vi "mediaBalls_v2.vi"(11 "Array Ball Pose + CamID":T1(array[cluster])) -> (3 "Ball out":cluster{"x":dbl, "y":dbl})   [LabVIEW 2018]
panel:
  in  "cluster":cluster{"x":dbl, "y":dbl}
  in  "Field Size 2":T2
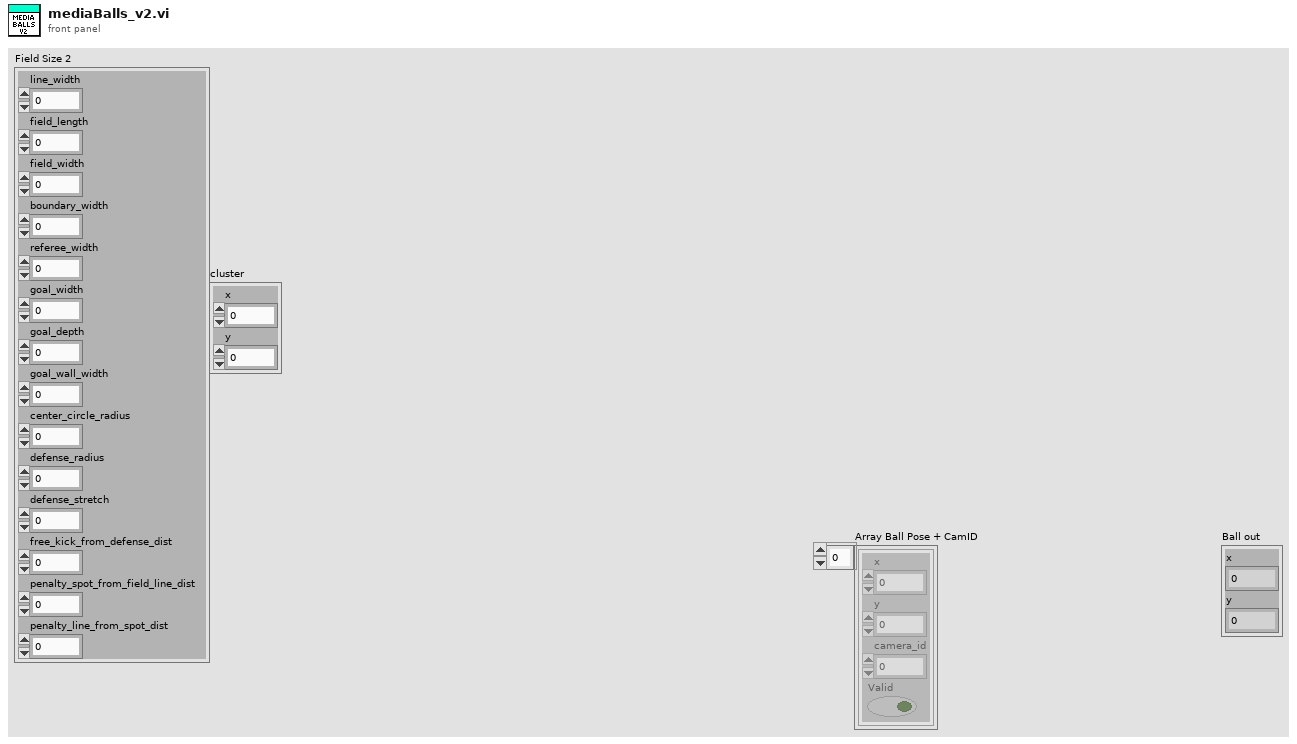
[diagram p1: front panel]
types:
  T1 = cluster{"x":sgl, "y":sgl, "camera_id":u32, "Valid":bool}[]
  T2 = cluster{"line_width":u32, "field_length":u32, "field_width":u32, "boundary_width":u32, "referee_width":u32, "goal_width":u32, "goal_depth":u32, "goal_wall_width":u32, "center_circle_radius":u32, "defense_radius":u32, "defense_stretch":u32, "free_kick_from_defense_dist":u32, "penalty_spot_from_field_line_dist":u32, "penalty_line_from_spot_dist":u32}
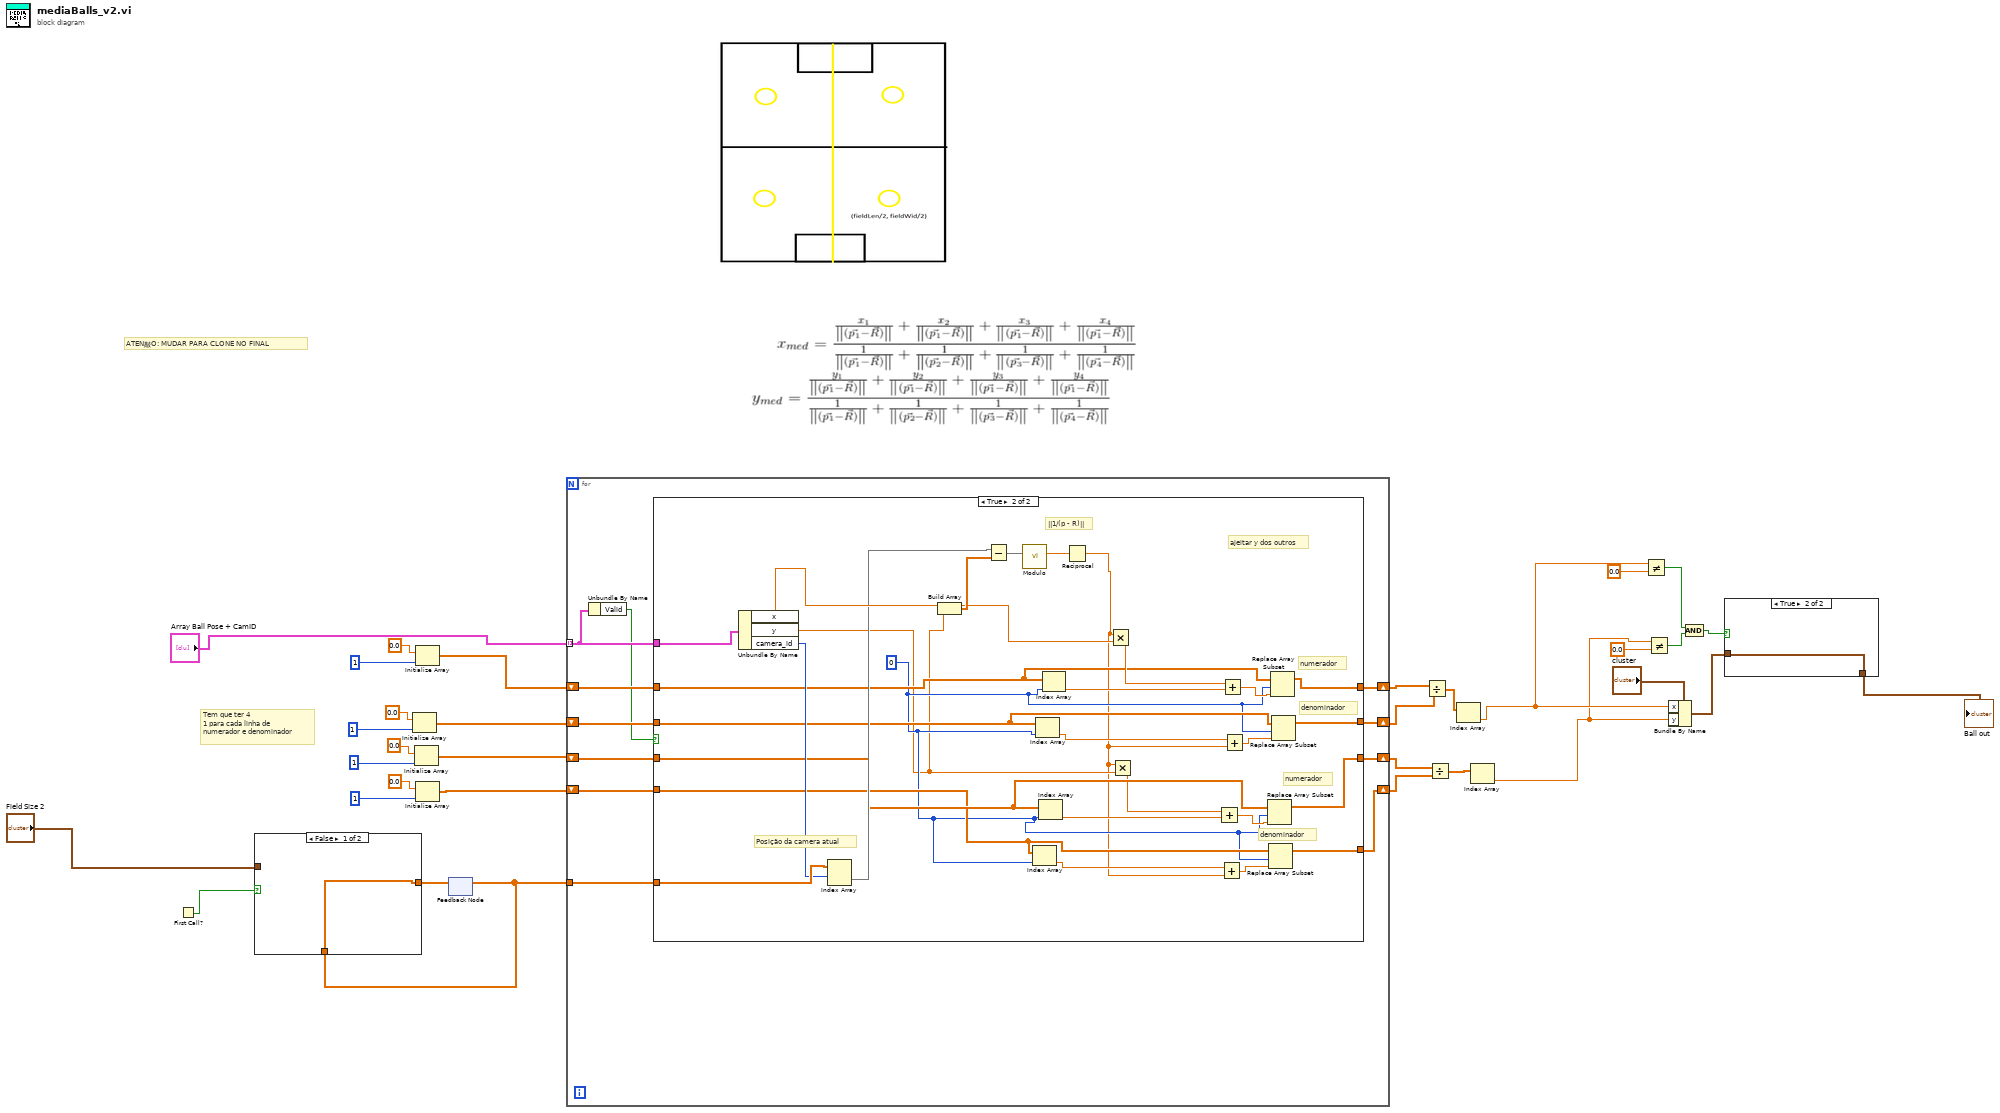
[diagram p0: block diagram]
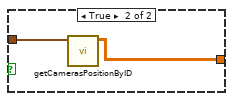
[diagram p2: hidden frame]
diagram:
  # "Tem que ter 4\n1 para cada linha de\nnumerador e denominador"
  # "ATEN敲O: MUDAR PARA CLONE NO FINAL"
  n1 = First Call?() -> (First Call?: T/F=w3:bool)
  n2 = Initialize Array(0.0 ("element"), 1 ("dimension size")) -> (w24:dbl[])
  n3 = Initialize Array(0.0 ("element"), 1 ("dimension size")) -> (w23:dbl[])
  n4 = Initialize Array(0.0 ("element"), 1 ("dimension size")) -> (w25:dbl[])
  n5 = Initialize Array(0.0 ("element"), 1 ("dimension size")) -> (w22:dbl[])
  n6 = feedback #1() -> (w1:dbl[][])  [unwired: 1 in]
  n7 = case shown="False" w3 {
    tunnel: "Field Size 2" -> [_ w36]
    tunnel: [w34 w35] -> w2
    tunnel: w1 -> [w34 _]
    frame False {
    }
    frame True {
      n8 = call "getCamerasPositionByID.vi"("Field Size 2"=w36) -> ("Cameras Positions"=w35:dbl[][])  [unwired: 10 in]
    }
  }
  n9 = feedback-in #1(w2) -> ()
  n10 = for {
    tunnel: "Array Ball Pose + CamID" -> [w38] mode=indexing
    tunnel: w1 -> [w47]
    shift-right: [w46] -> w21
    shift-left: w25 -> [w40]
    shift-right: [w45] -> w20
    shift-left: w24 -> [w39]
    shift-right: [w44] -> w19
    shift-left: w23 -> [w42]
    shift-right: [w43] -> w18
    shift-left: w22 -> [w41]
    n11 = Unbundle By Name(w38) -> ("Valid"=w37:bool)
    n12 = case shown="True" w37 {
      tunnel: w47 -> [_ w80]
      tunnel: [w51 w64] -> w46
      tunnel: [w50 w63] -> w45
      tunnel: [w49 w62] -> w44
      tunnel: [w48 w61] -> w43
      tunnel: w42 -> [w49 w60]
      tunnel: w41 -> [w48 w59]
      tunnel: w40 -> [w51 w58]
      tunnel: w39 -> [w50 w57]
      tunnel: w38 -> [_ w53]
      frame False {
      }
      frame True {
        w56 = 0 ("index")
        # "ajeitar y dos outros"
        # "denominador"
        # "numerador"
        # "denominador"
        # "numerador"
        # "||1/(p - R)||"
        # "Posição da camera atual"
        n13 = Unbundle By Name(w53) -> ("x"=w70:sgl, "y"=w55:sgl, "camera_id"=w79:u32)
        n14 = Index Array(array=w80, index (row)=w79) -> (element=w69:dbl[])  [unwired: 1 in]
        n15 = Build Array(w70, w55) -> (w78:sgl[])
        n16 = Subtract(x=w69, y=w78) -> (x-y=w77:dbl[])
        n17 = call "Modulo.vi"("2D vector"=w77) -> ("Modulo"=w76:dbl)  [unwired: 10 in]
        n18 = Index Array(array=w59, index=w56) -> (element=w65:dbl)
        n19 = Index Array(array=w57, index=w56) -> (element=w67:dbl)
        n20 = Index Array(array=w60, index=w56) -> (element=w66:dbl)
        n21 = Index Array(array=w58, index=w56) -> (element=w68:dbl)
        n22 = Reciprocal(x=w76) -> (1/x=w52:dbl)
        n23 = Multiply(x=w52, y=w70) -> (x*y=w75:dbl)
        n24 = Multiply(x=w52, y=w55) -> (x*y=w54:dbl)
        n25 = Add(x=w54, y=w66) -> (x+y=w72:dbl)
        n26 = Add(x=w65, y=w52) -> (x+y=w71:dbl)
        n27 = Add(x=w75, y=w68) -> (x+y=w74:dbl)
        n28 = Add(x=w67, y=w52) -> (x+y=w73:dbl)
        n29 = Replace Array Subset(array=w60, new element=w72, index=w56) -> (w62:dbl[])
        n30 = Replace Array Subset(array=w59, new element=w71, index=w56) -> (w61:dbl[])
        n31 = Replace Array Subset(array=w58, new element=w74, index=w56) -> (w64:dbl[])
        n32 = Replace Array Subset(array=w57, new element=w73, index=w56) -> (w63:dbl[])
      }
    }
  }
  n33 = Divide(x=w21, y=w20) -> (x/y=w10:dbl[])
  n34 = Divide(x=w19, y=w18) -> (x/y=w8:dbl[])
  n35 = Index Array(array=w10) -> (element=w9:dbl)  [unwired: 1 in]
  n36 = Index Array(array=w8) -> (element=w7:dbl)  [unwired: 1 in]
  n37 = Not Equal?(x=w9, y=0.0) -> (x != y?=w15:bool)
  n38 = Not Equal?(x=w7, y=0.0) -> (x != y?=w14:bool)
  n39 = Bundle By Name(cluster="cluster", "x"=w9, "y"=w7) -> (w12:cluster{"x":dbl, "y":dbl})
  n40 = And(x=w15, y=w14) -> (x .and. y?=w13:bool)
  n41 = case shown="True" w13 {
    tunnel: [w81 w82] -> w6
    tunnel: w12 -> [w81 w82]
    frame False {
    }
    frame True {
    }
  }
  "Ball out" <- w6
